vi "Page_MissingFiles.vi"(8 "error in":errorcluster, 10 "Missing Files":string[](array[string])) -> (0 "error out":errorcluster)   [LabVIEW 2010]
panel:
  out "Missing Files":string[][](table)
  in  "OK Button":bool
  # "The following files were not found based on the paths currently defined under System Configuration.\nPlease make sure the System Configuration points to the correct folders."
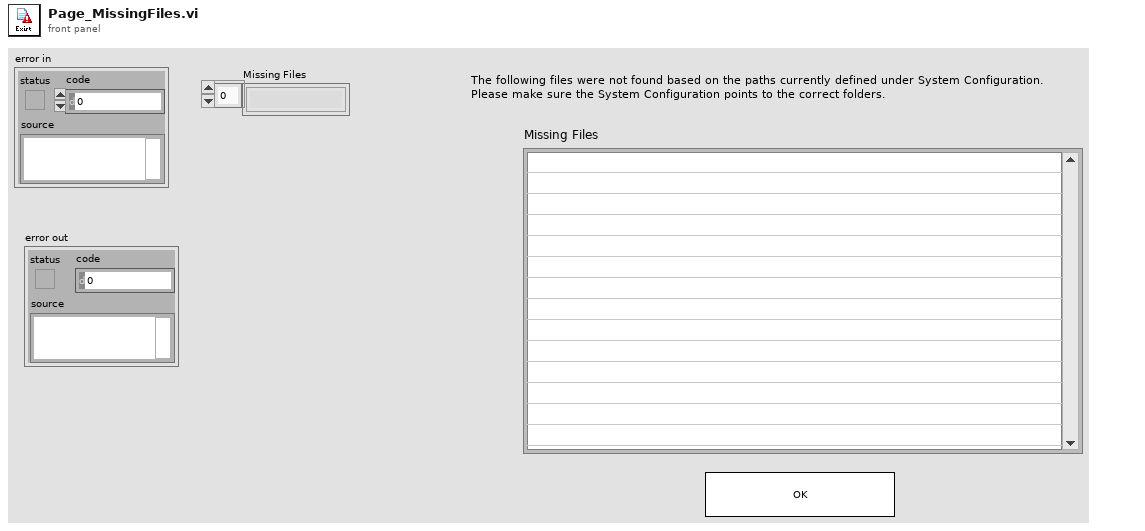
[diagram p1: front panel]
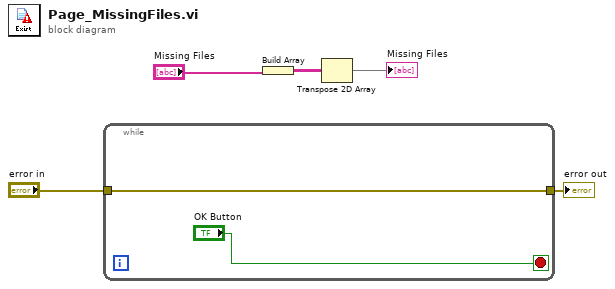
[diagram p0: block diagram]
diagram:
  n1 = while {
    tunnel: "error in" -> [w6]
    tunnel: [w6] -> w3
    stop <- "OK Button" stop-if-true
  }
  "error out" <- w3
  n2 = Build Array("Missing Files") -> (w5:string[][])
  n3 = Transpose 2D Array(2D array=w5) -> (transposed array=→"Missing Files":string[][])
